vi "Test Analysis API.vi"() -> ()   [LabVIEW 2019]
doc: "Analysis API Tester."
uses:
  Main UI Shared/Decimation input --cluster.ctl
  <vilib>/Utility/error.llb/DialogType.ctl
  Analysis.lvlib
  Filepath Editor/Filepath Editor.lvlib
  Main UI Shared/MAIN UI Shared.lvlib
panel:
  in  "Ch Datum":waveform(dbl)[](array[waveform])
  out "Data":cluster{"X":dbl[], "Y":dbl[]}[](graph)
  in  "Tau Delay (ms)":dbl
  in  "Contact":T1={"Contact stat?"=TRUE, "Contact Spread of dev"=0.0} {"Contact Spread of dev" format="%#_13g"}
  in  "Decimation":T2={"App"={"Dec"=1, "apply"=FALSE}, "Con"={"Dec"=1, "apply"=FALSE}, "Ret"={"Dec"=1, "apply"=FALSE}}
  in  "Savitzksky-Golay":T3={"Sidepoints (M)"=20.0, "Filter Order"=5} {"Filter Order" scale=0.0..10.0; "Sidepoints (M)" scale=0.0..10.0}
  in  "Update analysis parameters":bool
  in  "Show Diagram on Init":bool
  in  "Settings":bool
  out "error out":errorcluster
  in  "Stop Acquiring":bool
  in  "Start Acquiring":bool
  in  "Show Block Diagram":bool
  in  "Stop Module":bool
  in  "Start Module":bool
  in  "Hide Module Panel":bool
  in  "Show Module Panel":bool
  out "Status":string
  out "Module Running?":bool
  # "This VI tests the API for the Module."
  # "Contact"
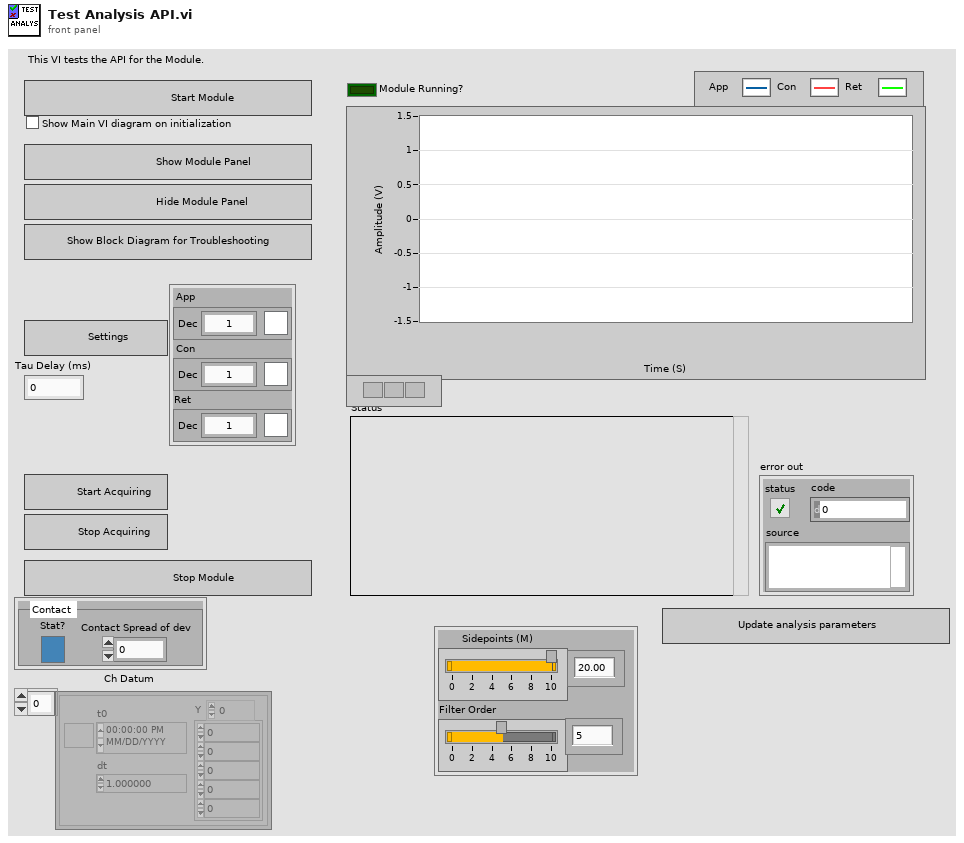
[diagram p1: front panel]
types:
  T1 = cluster{"Contact stat?":bool, "Contact Spread of dev":dbl}
  T2 = typedef "MAIN UI Shared.lvlib/Decimation input --cluster.ctl" = cluster{"App":cluster{"Dec":i32, "apply":bool}, "Con":cluster{"Dec":i32, "apply":bool}, "Ret":cluster{"Dec":i32, "apply":bool}}
  T3 = cluster{"Sidepoints (M)":dbl, "Filter Order":i32}
  T4 = typedef "Analysis.lvlib/Broadcast Events--cluster.ctl" = cluster{"Module Did Init":refnum<user-event>, "Status Updated":refnum<user-event>, "Error Reported":refnum<user-event>, "Module Did Stop":refnum<user-event>, "Update Module Execution Status":refnum<user-event>, "Fcurve sorted":refnum<user-event>}
  T5 = typedef "DialogType.ctl" = u16
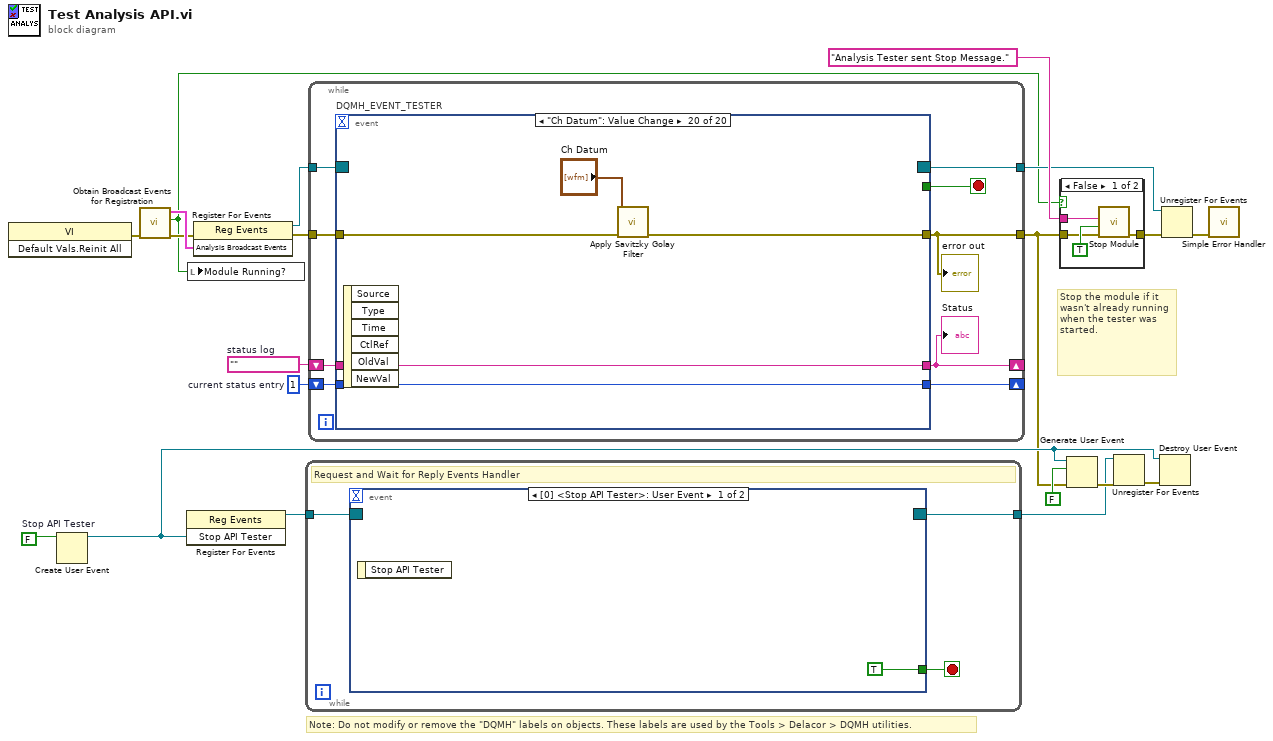
[diagram p0: block diagram]
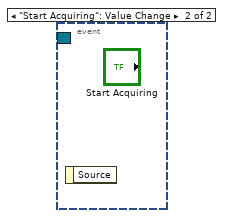
[diagram p2: hidden frame]
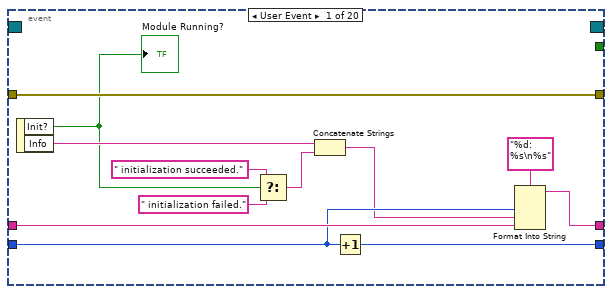
[diagram p3: hidden frame]
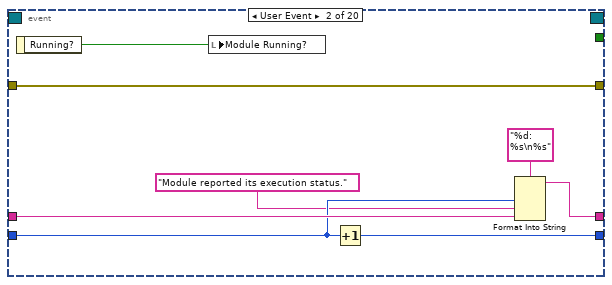
[diagram p4: hidden frame]
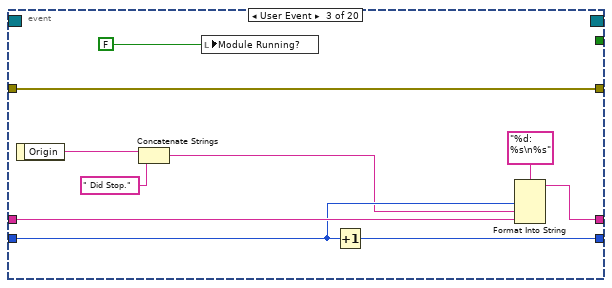
[diagram p5: hidden frame]
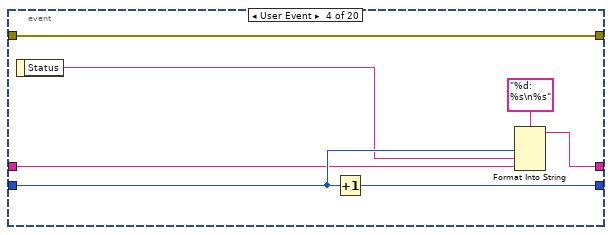
[diagram p6: hidden frame]
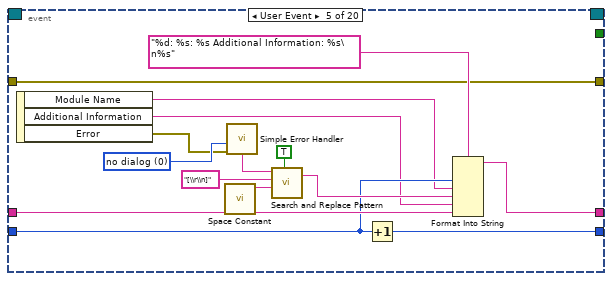
[diagram p7: hidden frame]
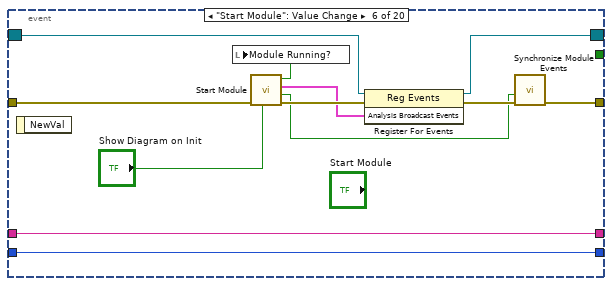
[diagram p8: hidden frame]
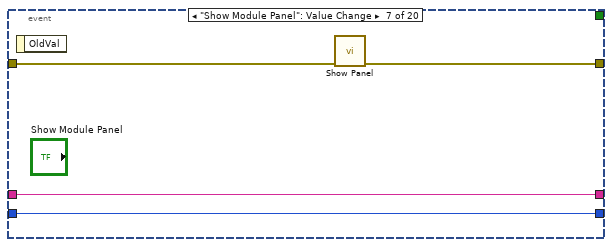
[diagram p9: hidden frame]
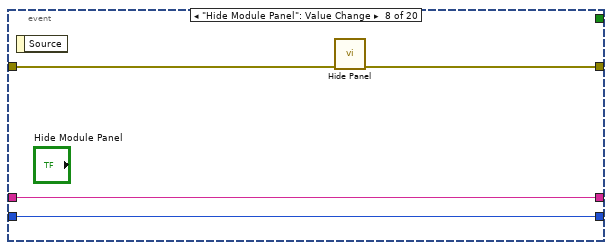
[diagram p10: hidden frame]
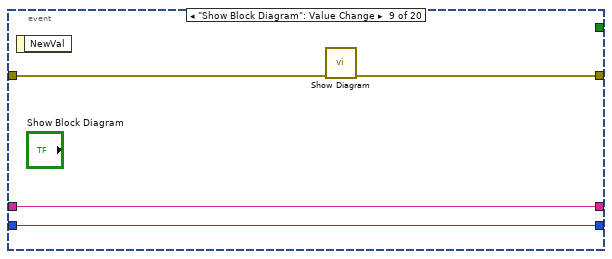
[diagram p11: hidden frame]
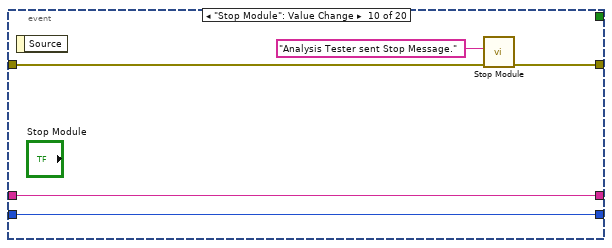
[diagram p12: hidden frame]
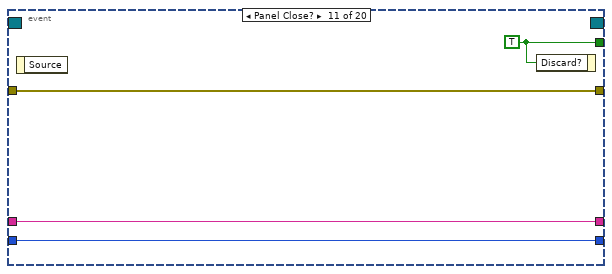
[diagram p13: hidden frame]
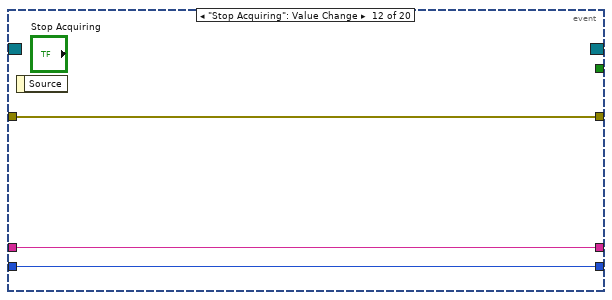
[diagram p14: hidden frame]
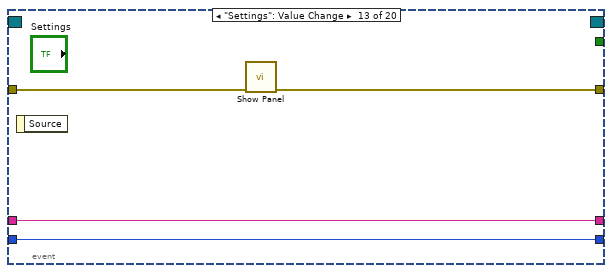
[diagram p15: hidden frame]
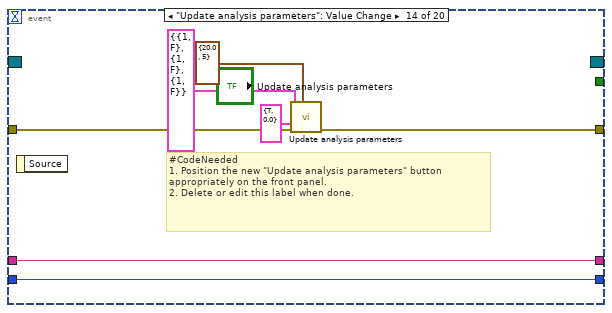
[diagram p16: hidden frame]
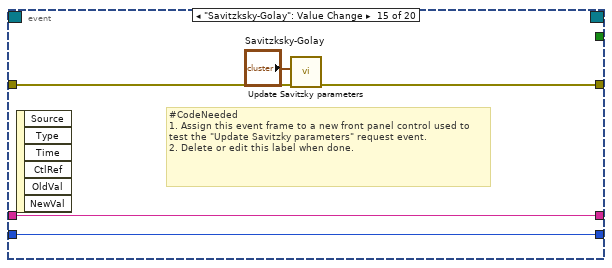
[diagram p17: hidden frame]
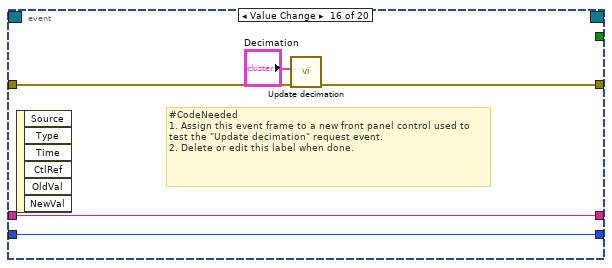
[diagram p18: hidden frame]
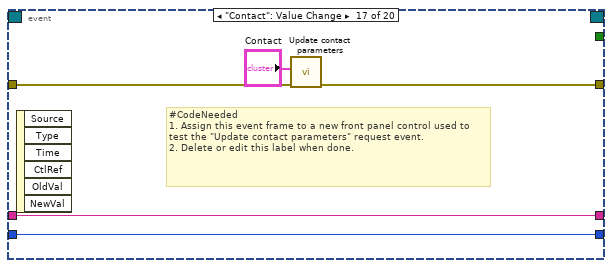
[diagram p19: hidden frame]
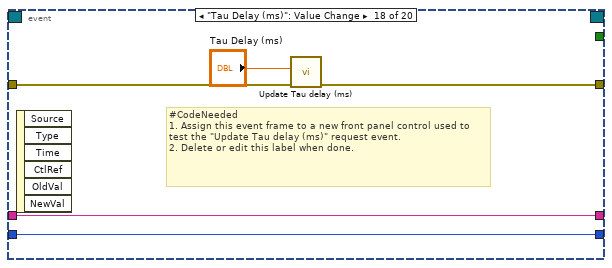
[diagram p20: hidden frame]
diagram:
  w10 = FALSE  # Stop API Tester
  w17 = 1  # current status entry
  w18 = ""  # status log
  # "Stop the module if it wasn't already running when the tester was started."
  # "Note: Do not modify or remove the \"DQMH\" labels on objects. These labels are used by the Tools > Delacor > DQMH utilities."
  n1 = invoke on="Invoke Node" class="VI" method="Default Vals.Reinit All"() -> (error out=w12:errorcluster)  [unwired: 3 in, 2 out]
  n2 = Create User Event(user event datatype=w10) -> (user event=w4:refnum<user-event>)  [unwired: 1 in, 1 out]
  n3 = call "Obtain Broadcast Events for Registration.vi"("error in"=w12) -> ("error out"=w11:errorcluster, "Already running?"=w3:bool, "Analysis Broadcast Events"=w15:T4)  [unwired: 8 in]
  n4 = register-events(w4) -> (reference out=w9:refnum<event-registration>)  [unwired: 2 in, 1 out]
  n5 = local write "Module Running?"(w3) -> ()
  n6 = register-events(error in=w11, w15) -> (reference out=w14:refnum<event-registration>, error out=w16:errorcluster)  [unwired: 1 in]
  n7 = while {
    tunnel: w9 -> [w23]
    tunnel: [w21] -> w6
    stop <- w22 stop-if-true
    # "Request and Wait for Reply Events Handler"
    n8 = event shown="[0] <Stop API Tester>: User Event" {
      selector: w23 -> [_ _]
      dyn-events: [_ _] -> w21
      timeout: _ -> [_ _]
      tunnel: [TRUE _] -> w22
      event User Event {
        n9 = event-data() -> ()  [unwired: 1 in, 1 out]
      }
      event "Start Acquiring": Value Change {
        n10 = event-data() -> ()  [unwired: 1 in, 1 out]
      }
    }
  }
  n11 = while {
    tunnel: w14 -> [w33]
    tunnel: [w26] -> w2
    shift-right: [w29] -> _
    shift-left: w18 -> [w31]
    shift-right: [w30] -> _
    shift-left: w17 -> [w32]
    tunnel: w16 -> [w28]
    tunnel: [w27] -> w13
    stop <- w25 stop-if-true
    n12 = event "DQMH_EVENT_TESTER" shown="[19] \"Ch Datum\": Value Change" {
      selector: w33 -> [_ _ _ _ _ w91 _ _ _ _ _ _ _ _ _ _ _ _ _ _]
      dyn-events: [_ _ _ _ _ w90 _ _ _ _ _ _ _ _ _ _ _ _ _ _] -> w27
      timeout: _ -> [_ _ _ _ _ _ _ _ _ _ _ _ _ _ _ _ _ _ _ _]
      tunnel: [_ _ _ _ _ _ _ _ _ _ w118 _ _ _ _ _ _ _ _ _] -> w25
      tunnel: [w45 w47 w54 w64 w74 w89 w101 w105 w106 w112 w115 w121 w122 w129 w134 w139 w144 w149 w162 w164] -> w26
      tunnel: w32 -> [w42 w51 w61 w67 w77 w94 w99 w103 w107 w113 w116 w119 w124 w130 w135 w140 w145 w150 w159 w165]
      tunnel: w31 -> [w43 w52 w62 w66 w78 w95 w100 w104 w108 w114 w117 w120 w125 w131 w136 w141 w146 w151 w161 w166]
      tunnel: [w40 w49 w59 w68 w75 w95 w100 w104 w108 w114 w117 w120 w125 w131 w136 w141 w146 w151 w160 w166] -> w29
      tunnel: [w41 w50 w60 w70 w76 w94 w99 w103 w107 w113 w116 w119 w124 w130 w135 w140 w145 w150 w158 w165] -> w30
      tunnel: w28 -> [w45 w47 w54 w64 w74 w88 w98 w102 w109 w110 w115 w121 w123 w132 w137 w142 w147 w152 w162 w167]
      event User Event {
        n13 = event-data() -> ("Init?"=w37:bool, "Info"=w39:string)  [unwired: 1 in]
        "Module Running?" <- w37
        n14 = Select(t=" initialization succeeded.", s=w37, f=" initialization failed.") -> (s? t:f=w34:string)
        n15 = Concatenate Strings(w39, w34) -> (w38:string)
        n16 = Increment(x=w42) -> (x+1=w41:i32)
        n17 = Format Into String(format string="%d: %s\n%s", w42, w38, w43) -> (resulting string=w40:string)  [unwired: 2 in, 1 out]
      }
      event User Event {
        n18 = event-data() -> ("Running?"=w46:bool)  [unwired: 1 in]
        n19 = local write "Module Running?"(w46) -> ()
        n20 = Increment(x=w51) -> (x+1=w50:i32)
        n21 = Format Into String(format string="%d: %s\n%s", w51, "Module reported its execution status.", w52) -> (resulting string=w49:string)  [unwired: 2 in, 1 out]
      }
      event User Event {
        n22 = event-data() -> ("Origin"=w58:string)  [unwired: 1 in]
        n23 = Concatenate Strings(w58, " Did Stop.") -> (w57:string)
        n24 = local write "Module Running?"(FALSE ("Module Did Init?")) -> ()
        n25 = Increment(x=w61) -> (x+1=w60:i32)
        n26 = Format Into String(format string="%d: %s\n%s", w61, w57, w62) -> (resulting string=w59:string)  [unwired: 2 in, 1 out]
      }
      event User Event {
        n27 = event-data() -> ("Status"=w65:string)  [unwired: 1 in]
        n28 = Increment(x=w67) -> (x+1=w70:i32)
        n29 = Format Into String(format string="%d: %s\n%s", w67, w65, w66) -> (resulting string=w68:string)  [unwired: 2 in, 1 out]
      }
      event User Event {
        w79 = T5 0 items=["no dialog", "OK message", "continue or stop message", "OK message + warnings", "continue/stop + warnings"] ("type of dialog (OK msg:1)")
        n30 = event-data() -> ("Module Name"=w73:string, "Additional Information"=w72:string, "Error"=w71:errorcluster)  [unwired: 1 in]
        n31 = call <vilib>:"Space Constant.vi"() -> ("String"=w83:string)
        n32 = call <vilib>:"Simple Error Handler.vi"("type of dialog (OK msg:1)"=w79, "error in (no error)"=w71) -> ("message"=w80:string)  [unwired: 3 in, 4 out]
        n33 = call <vilib>:"Search and Replace Pattern.vi"("string"=w80, "regular expression (\"\")"="[\\r\\n]" ("regular expression (\"\")"), "replace string (\"\")"=w83, "replace all? (F)"=TRUE ("replace all CR/LF with spaces")) -> ("result string"=w81:string)  [unwired: 1 in, 1 out]
        n34 = Increment(x=w77) -> (x+1=w76:i32)
        n35 = Format Into String(format string="%d: %s: %s Additional Information: %s\n%s", w77, w73, w81, w72, w78) -> (resulting string=w75:string)  [unwired: 2 in, 1 out]
      }
      event "Start Module": Value Change {
        n36 = event-data() -> ()  [unwired: 1 in, 1 out]
        n37 = call "Start Module.vi"("Show Main VI Diagram on Init (F)"="Show Diagram on Init", "error in"=w88) -> ("error out"=w96:errorcluster, "Wait for Event Sync?"=w93:bool, "Analysis Broadcast Events"=w92:T4, "Module Was Already Running?"=w87:bool)  [unwired: 6 in]
        n38 = local write "Module Running?"(w87) -> ()
        n39 = register-events(reference=w91, error in=w96, w92) -> (reference out=w90:refnum<event-registration>, error out=w97:errorcluster)
        n40 = call "Synchronize Module Events.vi"("error in (no error)"=w97, "Wait for Event Sync?"=w93) -> ("error out"=w89:errorcluster)  [unwired: 9 in]
      }
      event "Show Module Panel": Value Change {
        n41 = event-data() -> ()  [unwired: 1 in, 1 out]
        n42 = call "Show Panel.vi"("error in (no error)"=w98) -> ("error out"=w101:errorcluster)  [unwired: 10 in]
      }
      event "Hide Module Panel": Value Change {
        n43 = event-data() -> ()  [unwired: 1 in, 1 out]
        n44 = call "Hide Panel.vi"("error in (no error)"=w102) -> ("error out"=w105:errorcluster)  [unwired: 10 in]
      }
      event "Show Block Diagram": Value Change {
        n45 = event-data() -> ()  [unwired: 1 in, 1 out]
        n46 = call "Show Diagram.vi"("error in (no error)"=w109) -> ("error out"=w106:errorcluster)  [unwired: 10 in]
      }
      event "Stop Module": Value Change {
        n47 = event-data() -> ()  [unwired: 1 in, 1 out]
        n48 = call "Stop Module.vi"("error in"=w110, "Origin"="Analysis Tester sent Stop Message.") -> ("error out"=w112:errorcluster)  [unwired: 9 in]
      }
      event Panel Close? {
        w118 = TRUE ("Discard?")
        n49 = event-data() -> ()  [unwired: 1 in, 1 out]
        n50 = event-data ("Event Filter Node")("Discard?"=w118) -> ()  [unwired: 1 in, 1 out]
      }
      event "Stop Acquiring": Value Change {
        n51 = event-data() -> ()  [unwired: 1 in, 1 out]
      }
      event "Settings": Value Change {
        n52 = event-data() -> ()  [unwired: 1 in, 1 out]
        n53 = call "Show Panel.vi"("error in (no error)"=w123) -> ("error out"=w122:errorcluster)  [unwired: 10 in]
      }
      event "Update analysis parameters": Value Change {
        # "#CodeNeeded\n1. Position the new \"Update analysis parameters\" button appropriately on the front panel.\n2. Delete or edit this label when done."
        n54 = event-data() -> ()  [unwired: 1 in, 1 out]
        n55 = call "Update analysis parameters.vi"("Savitzksky-Golay"=T3 {"Sidepoints (M)"=20.0, "Filter Order"=5}, "error in"=w132, "Decimation"=T2 {"App"={"Dec"=1, "apply"=FALSE}, "Con"={"Dec"=1, "apply"=FALSE}, "Ret"={"Dec"=1, "apply"=FALSE}}, "Contact"=T1 {"Contact stat?"=TRUE, "Contact Spread of dev"=0.0}) -> ("error out"=w129:errorcluster)  [unwired: 5 in, 2 out]
      }
      event "Savitzksky-Golay": Value Change {
        # "#CodeNeeded\n1. Assign this event frame to a new front panel control used to test the \"Update Savitzky parameters\" request event.\n2. Delete or edit this label when done."
        n56 = event-data() -> ()  [unwired: 1 in, 6 out]
        n57 = call "Update Savitzky parameters.vi"("error in"=w137, "Savitzksky-Golay"="Savitzksky-Golay") -> ("error out"=w134:errorcluster)  [unwired: 9 in]
      }
      event Value Change {
        # "#CodeNeeded\n1. Assign this event frame to a new front panel control used to test the \"Update decimation\" request event.\n2. Delete or edit this label when done."
        n58 = event-data() -> ()  [unwired: 1 in, 6 out]
        n59 = call "Update decimation.vi"("error in"=w142, "Decimation"="Decimation") -> ("error out"=w139:errorcluster)  [unwired: 9 in]
      }
      event "Contact": Value Change {
        # "#CodeNeeded\n1. Assign this event frame to a new front panel control used to test the \"Update contact parameters\" request event.\n2. Delete or edit this label when done."
        n60 = event-data() -> ()  [unwired: 1 in, 6 out]
        n61 = call "Update contact parameters.vi"("error in"=w147, "Contact"="Contact") -> ("error out"=w144:errorcluster)  [unwired: 9 in]
      }
      event "Tau Delay (ms)": Value Change {
        # "#CodeNeeded\n1. Assign this event frame to a new front panel control used to test the \"Update Tau delay (ms)\" request event.\n2. Delete or edit this label when done."
        n62 = event-data() -> ()  [unwired: 1 in, 6 out]
        n63 = call "Update Tau delay (ms).vi"("error in"=w152, "Tau Delay (ms)"="Tau Delay (ms)") -> ("error out"=w149:errorcluster)  [unwired: 9 in]
      }
      event User Event {
        # "#CodeNeeded\n1. Process the event data sent by the \"Fcurve sorted\" broadcast event.\n2. Delete or edit this label when done."
        n64 = event-data() -> ("Fcurve out"=→"Data":cluster{"X":dbl[], "Y":dbl[]}[])  [unwired: 1 in]
        n65 = Format Into String(format string="Response Received - %s", "Fcurve recieved" ("input 1")) -> (resulting string=w155:string)  [unwired: 2 in, 1 out]
        n66 = Increment(x=w159) -> (x+1=w158:i32)
        n67 = Format Into String(format string="%d: %s\n%s", w159, w155, w161) -> (resulting string=w160:string)  [unwired: 2 in, 1 out]
      }
      event "Ch Datum": Value Change {
        n68 = event-data() -> ()  [unwired: 1 in, 6 out]
        n69 = call "Apply Savitzky Golay Filter.vi"("error in"=w167, "Ch Datum"="Ch Datum") -> ("error out"=w164:errorcluster)  [unwired: 7 in, 2 out]
      }
    }
    "Status" <- w29
    "error out" <- w26
  }
  n70 = case shown="False" w3 {
    tunnel: [w171 w172] -> w20
    tunnel: "Analysis Tester sent Stop Message." ("Origin") -> [w170 _]
    tunnel: w2 -> [w168 w172]
    frame False {
      n71 = call "Stop Module.vi"("error in"=w168, "Wait for Module to Stop? (F)"=TRUE ("Wait for Module to stop?"), "Origin"=w170) -> ("error out"=w171:errorcluster)  [unwired: 8 in]
    }
    frame True {
    }
  }
  n72 = Generate User Event(user event=w4, event data cluster=FALSE ("Stop API Tester"), error in=w2) -> (error out=w7:errorcluster)  [unwired: 1 in, 1 out]
  n73 = Unregister For Events(event registration refnum=w6, error in=w7) -> (error out=w5:errorcluster)
  n74 = Destroy User Event(user event=w4, error in=w5) -> ()  [unwired: 1 out]
  n75 = Unregister For Events(event registration refnum=w13, error in=w20) -> (error out=w1:errorcluster)
  n76 = call <vilib>:"Simple Error Handler.vi"("error in (no error)"=w1) -> ()  [unwired: 4 in, 5 out]
